vi "Set_TDMS_Properties.vi"(11 "Total time":dbl) -> (3 "TDMS Properties":string[](array[string]))   [LabVIEW 2015]
uses:
  MARS_Global_var.vi
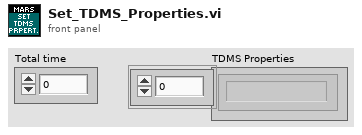
[diagram p1: front panel]
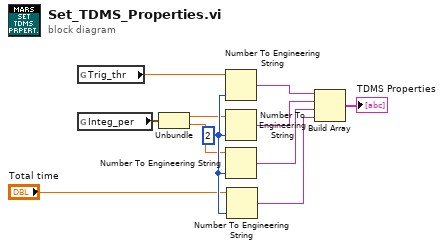
[diagram p0: block diagram]
diagram:
  w6 = i16 2 ("precision (6)")
  n1 = global read "MARS_Global_var.vi" "Trig_thr"() -> (w4:dbl)
  n2 = global read "MARS_Global_var.vi" "Integ_per"() -> (w1:cluster{dbl, dbl})
  n3 = Unbundle(w1) -> (w2:dbl, w3:dbl)
  n4 = Number To Engineering String(2:w6, 4:w4) -> (0:w7:string)  [unwired: 2 in]
  n5 = Number To Engineering String(2:w6, 4:w2) -> (0:w8:string)  [unwired: 2 in]
  n6 = Number To Engineering String(2:w6, 4:w3) -> (0:w9:string)  [unwired: 2 in]
  n7 = Number To Engineering String(2:w6, 4:"Total time") -> (0:w10:string)  [unwired: 2 in]
  n8 = Build Array(w7, w8, w9, w10) -> (→"TDMS Properties":string[])
